vi "SL TAGS Close.vi"(8 "error in (no error)":errorcluster, 10 "Tag Type":T1, 11 "EEISysLink in":refnum<class "EEISysLink.lvclass">) -> (0 "error out":errorcluster, 3 "EEISysLink out":refnum<class "EEISysLink.lvclass">)   [LabVIEW 2017, in "EEISysLink.lvclass"]
doc: "Close all tag instances of the specified type.\n\nJames Tillett\nEndeavor Engineering Inc.\nwww.endeavoreng.com"
uses:
  EEISysLink.lvclass
  Controls/SL Tag Type.ctl
  EEISysLink.lvclass/EEISysLink.ctl
  Controls/SL Tag.ctl
  Controls/SL Tag Properties.ctl
  Controls/SL Tag Data Type.ctl
  Controls/SL Tag Interpolation Method.ctl
  Controls/SL Tag Unit of Measure.ctl
  <vilib>/Skyline/Tag/Wrapper/Wrapper_class/NI Skyline Tag.lvclass
  <vilib>/Skyline/Tag/Shared/typedefs/Tag Cluster.ctl
  <vilib>/Skyline/Tag/Shared/typedefs/DataType.ctl
  <vilib>/Skyline/Tag/Wrapper/Wrapper_class/Close Tag (Single).vi
  <vilib>/Skyline/Tag/Shared/NI Skyline Tag.lvlib
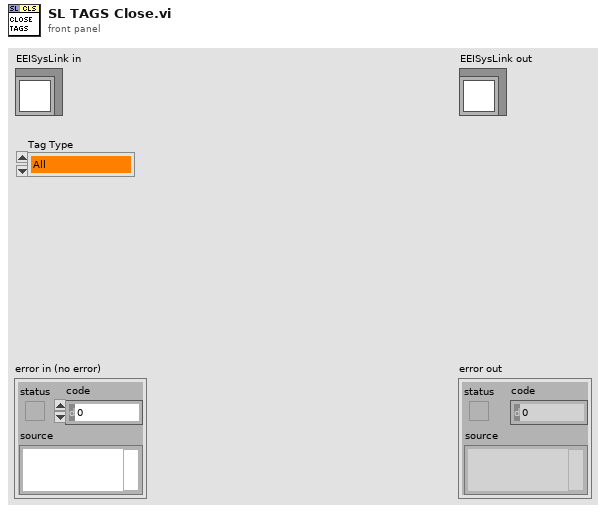
[diagram p1: front panel]
types:
  T1 = typedef "EEISysLink.lvclass/SL Tag Type.ctl" = enum16{"All", "Supervisor", "Worker"}
  T2 = typedef "EEISysLink.lvclass/SL Tag.ctl" = cluster{"Class Properties":T3, "SL Tag":refnum<class "NI Skyline Tag.lvclass">, "SystemLink Cluster":T7, "Class Value":variant}
  T3 = typedef "EEISysLink.lvclass/SL Tag Properties.ctl" = cluster{"Class Data Type":T4, "Name":string, "Description":string, "Interpolation Method":T5, "Unit of Measure":T6, "Maximum Interpolation":string, "Role":T1}
  T4 = typedef "EEISysLink.lvclass/SL Tag Data Type.ctl" = enum16{"Double", "Integer", "String", "Boolean", "Waveform"}
  T5 = typedef "EEISysLink.lvclass/SL Tag Interpolation Method.ctl" = enum16{"linear", "pilinear", "step"}
  T6 = typedef "EEISysLink.lvclass/SL Tag Unit of Measure.ctl" = enum16{"no units", "Second", "Hour", "Minute", "Day", "Year", "Month", "Week", "Foot", "Yard", "Meter", "Centimeter", "Inch", "Mile", "Nautical Mile", "Miles per Hour", "Meters per second", "Square meter", "Cubic meter", "Cubic centimeter", "Cubic inch", "Liter", "Gallon", "Gallons dry US", "Gallon UK", "Percent", "Revolutions per minute", "Revolution", "Degree angle", "Astronomical Unit", "Atom", "Atomic mass", "Bar", "Byte", "C (speed of light)", "Curie", "Decibel", "Electron Volt", "Ounce", "Knot", "G", "Grade", "Are", "Hectare", "Faraday", "Franklin", "Gilbert", "Erg", "Lambert", "Maxwell", "Gauss", "Electron mass", "Kilogram force", "Pound force", "Rad", "Centiradian", "Sphere", "Mach", "Fluid Ounces", "Fluid Ounces UK", "Fahrenheit", "Celsius", "Kelvin", "Rankine", "Gram", "Kilogram", "Pound", "Short/US Ton", "Long/UK ton", "Metric ton", "Mole", "Pounds per square inch", "Inches water column", "Torr", "Millitorr", "Millimeter mercury", "Inches mercury", "Bar (2)", "Atmosphere", "Pascal", "Watt", "kiloWatt", "Horsepower", "Kilowatt Hour", "British thermal units", "Millions of BTU", "Ampere", "Candela", "Radian", "Steradian", "Bit", "Hertz", "Newton", "Joule", "Coulomb", "Volt", "Farad", "Ohm", "Siemens", "Weber", "Tesla", "Henry", "Lumen", "Lux", "Becqueral", "Gray", "Sievert", "Katal", "Angstrom", "Light Year", "Parsec", "Point", "Pixel", "Dyne", "Kilogram force (2)", "Pound force (2)", "Rem", "Rutherford", "Roentgen"}
  T7 = typedef "NI Skyline Tag.lvlib/Tag Cluster.ctl" = cluster{"Path":string, "Data Type":T8, "Value":variant, "Time Stamp":timestamp}
  T8 = typedef "NI Skyline Tag.lvlib/DataType.ctl" = enum32{"Double", "Integer", "String"}
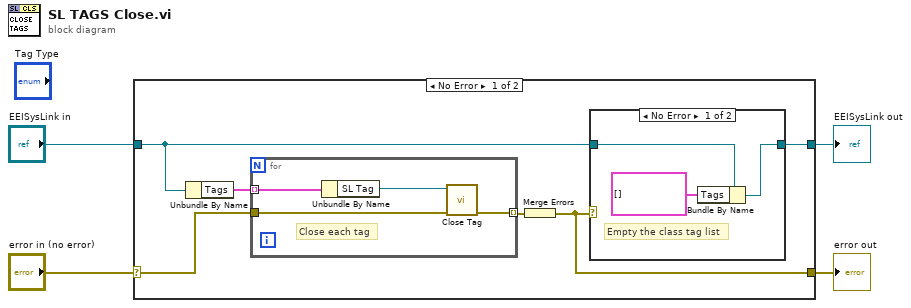
[diagram p0: block diagram]
diagram:
  n1 = case shown="No Error" "error in (no error)" {
    selector: "error in (no error)" -> [w8 w20]
    tunnel: [w7 w20] -> w3
    tunnel: [w5 w19] -> w1
    tunnel: "EEISysLink in" -> [w6 w19]
    frame No Error {
      n2 = Unbundle By Name(w6) -> ("Tags"=w10:T2[])
      n3 = for {
        tunnel: w10 -> [w18] mode=indexing
        tunnel: w8 -> [w16]
        tunnel: [w15] -> w9 mode=indexing
        # "Close each tag"
        n4 = Unbundle By Name(w18) -> ("SL Tag"=w17:refnum<class "NI Skyline Tag.lvclass">)
        n5 = call-poly <vilib>:"Close Tag.vi"("error in (no error)"=w16, "tag in"=w17) -> ("error out"=w15:errorcluster)  [unwired: 9 in]
      }
      n6 = Merge Errors(w9) -> (w7:errorcluster)
      n7 = case shown="No Error" w7 {
        tunnel: w6 -> [w13 w14]
        tunnel: [w11 w14] -> w5
        frame No Error {
          # "Empty the class tag list"
          n8 = Bundle By Name(cluster=w13, "Tags"=T2[] []) -> (w11:refnum<class "EEISysLink.lvclass">)
        }
        frame Error {
          # "Error so don't change tag list"
        }
      }
    }
    frame Error {
    }
  }
  "error out" <- w3
  "EEISysLink out" <- w1
